vi "calculate binning sub.vi"(9 "Y Resolution":i32, 10 "X Resolution":i32, 11 "MaxGuiPixel":dbl) -> (3 "GUIbinning":dbl)   [LabVIEW 2018]
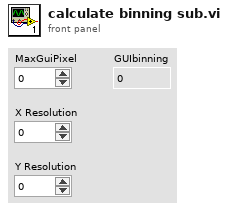
[diagram p1: front panel]
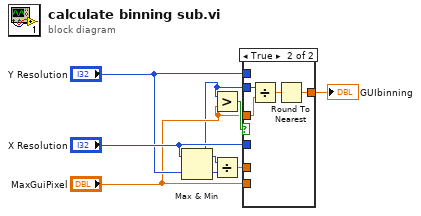
[diagram p0: block diagram]
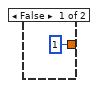
[diagram p2: hidden frame]
diagram:
  n1 = Max & Min(x="X Resolution", y="Y Resolution") -> (max(x,y)=w1:i32, min(x,y)=w8:i32)
  n2 = Greater?(x=w1, y="MaxGuiPixel") -> (0:w6:bool)
  n3 = Divide(x=w1, y=w8) -> (x/y=w7:dbl)
  n4 = case shown="True" w6 {
    tunnel: w7 -> [_ _]
    tunnel: "MaxGuiPixel" -> [_ _]
    tunnel: "X Resolution" -> [_ _]
    tunnel: "Y Resolution" -> [_ _]
    tunnel: [1 w12] -> w5
    tunnel: "MaxGuiPixel" -> [_ w11]
    tunnel: w1 -> [_ w10]
    frame False {
    }
    frame True {
      n5 = Divide(x=w10, y=w11) -> (x/y=w13:dbl)
      n6 = Round To Nearest(number=w13) -> (nearest integer value=w12:dbl)
    }
  }
  "GUIbinning" <- w5
